vi "file created event callback.vi"(4 "queue out":refnum<queue>, 5 "Event Data":cluster{"sender":refnum<k24>, "e":refnum<k24>}, 6 "Control Ref":refnum<k24>, 7 "Event Common Data":T1) -> ()   [LabVIEW 2020, in "FileCopyEventBased.lvclass"]
uses:
  FileCopyEventBased.lvclass
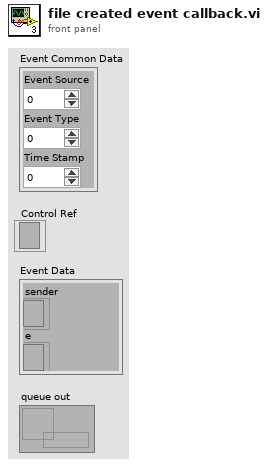
[diagram p1: front panel]
types:
  T1 = cluster{"Event Source":i32, "Event Type":u32, "Time Stamp":u32}
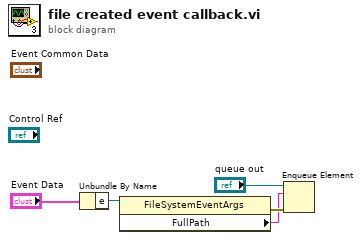
[diagram p0: block diagram]
diagram:
  n1 = Unbundle By Name("Event Data") -> ("e"=w3:refnum<k24>)
  n2 = property class="FileSystemEventArgs"(reference=w3) -> (error out=w5:errorcluster, "FullPath"=w2:string)  [unwired: 1 in, 1 out]
  n3 = Enqueue Element(queue="queue out", element=w2, error in (no error)=w5) -> ()  [unwired: 1 in, 3 out]
